vi "IRSensor(SubVI).vi"() -> (3 "interpolation value":dbl)   [LabVIEW 2017]
uses:
  <vilib>/Analysis/NI_AALPro.lvlib
  <vilib>/Analysis/NI_AALBase.lvlib
  <vilib>/Analysis/baseanly.llb/Mean (DBL).vi
  <vilib>/myRIO/Express VI/Onboard IO/AI/AI Express VI.xnode
  <vilib>/myRIO/Instrument Drivers/Onboard IO/AI/vis/Read.vi
  <vilib>/myRIO/Instrument Drivers/Onboard IO/AI/AI.lvlib
  <vilib>/myRIO/Common/Instrument Driver Framework/Utilities/typedefs/Analog Scaling Constants.ctl
  <vilib>/myRIO/Common/Instrument Driver Framework/Utilities/typedefs/Analog Scaling Constants List.ctl
  <vilib>/myRIO/Common/Instrument Driver Framework/myRIO v1.0/AI/typedefs/AI Channels Enum.ctl
  <vilib>/myRIO/Common/Instrument Driver Framework/myRIO v1.0/AI/typedefs/AI Channels List.ctl
  <vilib>/myRIO/Common/Instrument Driver Framework/Utilities/typedefs/Generic FPGA Reference.ctl
  <vilib>/myRIO/Common/Instrument Driver Framework/Utilities/typedefs/myRIO v1.0 Reference.ctl
  <vilib>/myRIO/Common/Instrument Driver Framework/Utilities/typedefs/Hardware Version Enum.ctl
  <vilib>/myRIO/Common/Instrument Driver Framework/Utilities/typedefs/myRIO Generic Hardware Reference.ctl
  <vilib>/myRIO/Instrument Drivers/Onboard IO/AI/typedefs/AI Reference.ctl
  <vilib>/myRIO/Instrument Drivers/Onboard IO/AI/vis/myRIO AI Open.xnode
  <vilib>/myRIO/Common/Instrument Driver Framework/Utilities/vis/Is FPGA Ref Available.vi
  <vilib>/myRIO/Common/Instrument Driver Framework/myRIO v1.0/AI/vis/myRIO v1.1 Open AI.vi
  <vilib>/userdefined/High Color/nirio_resource_hc.ctl
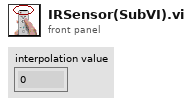
[diagram p1: front panel]
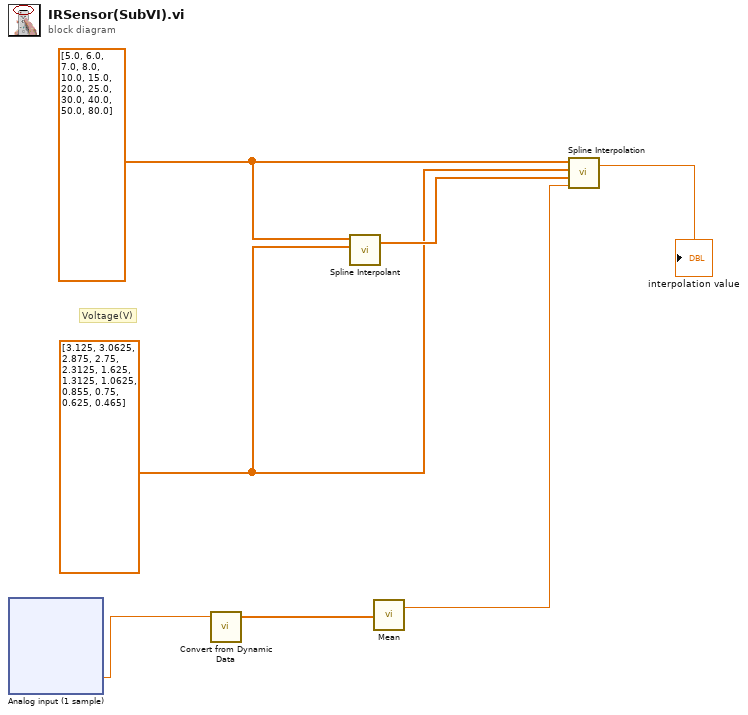
[diagram p0: block diagram]
diagram:
  w3 = dbl[] [5.0, 6.0, 7.0, 8.0, 10.0, 15.0, 20.0, 25.0, 30.0, 40.0, 50.0, 80.0]
  w4 = dbl[] [3.125, 3.0625, 2.875, 2.75, 2.3125, 1.625, 1.3125, 1.0625, 0.855, 0.75, 0.625, 0.465]
  # "Voltage(V)"
  n1 = xnode "Analog input (1 sample)"() -> ("B/AI0 (Pin 3)"=w1:dbl)  [unwired: 1 in, 1 out]
  n2 = call "Convert from Dynamic Data"("Dynamic Data Type"=w1) -> ("Array"=w2:dbl[])  [unwired: 3 in]
  n3 = call <vilib>:"Spline Interpolant.vi"("X"=w4, "Y"=w3) -> ("Interpolant"=w5:dbl[])  [unwired: 2 in, 1 out]
  n4 = call-poly <vilib>:"Mean.vi"("X"=w2) -> ("mean"=w6:dbl)  [unwired: 1 out]
  n5 = call <vilib>:"Spline Interpolation.vi"("x value"=w6, "Interpolant"=w5, "X"=w4, "Y"=w3) -> ("interpolation value"=→"interpolation value":dbl)  [unwired: 1 out]
